vi "CleanROIs (SubVI).vi"(2 "Image Pixels (U8) 2":u8[][](array[numeric]), 3 "ROI array out 3":u32[][](array[numeric])) -> (0 "ROI array out 2":u32[][](array[numeric]))   [LabVIEW 2011, in "OfflineTracker.lvlib"]
uses:
  OfflineTracker.lvlib
panel:
  out "Array":bool[](array[boolean])
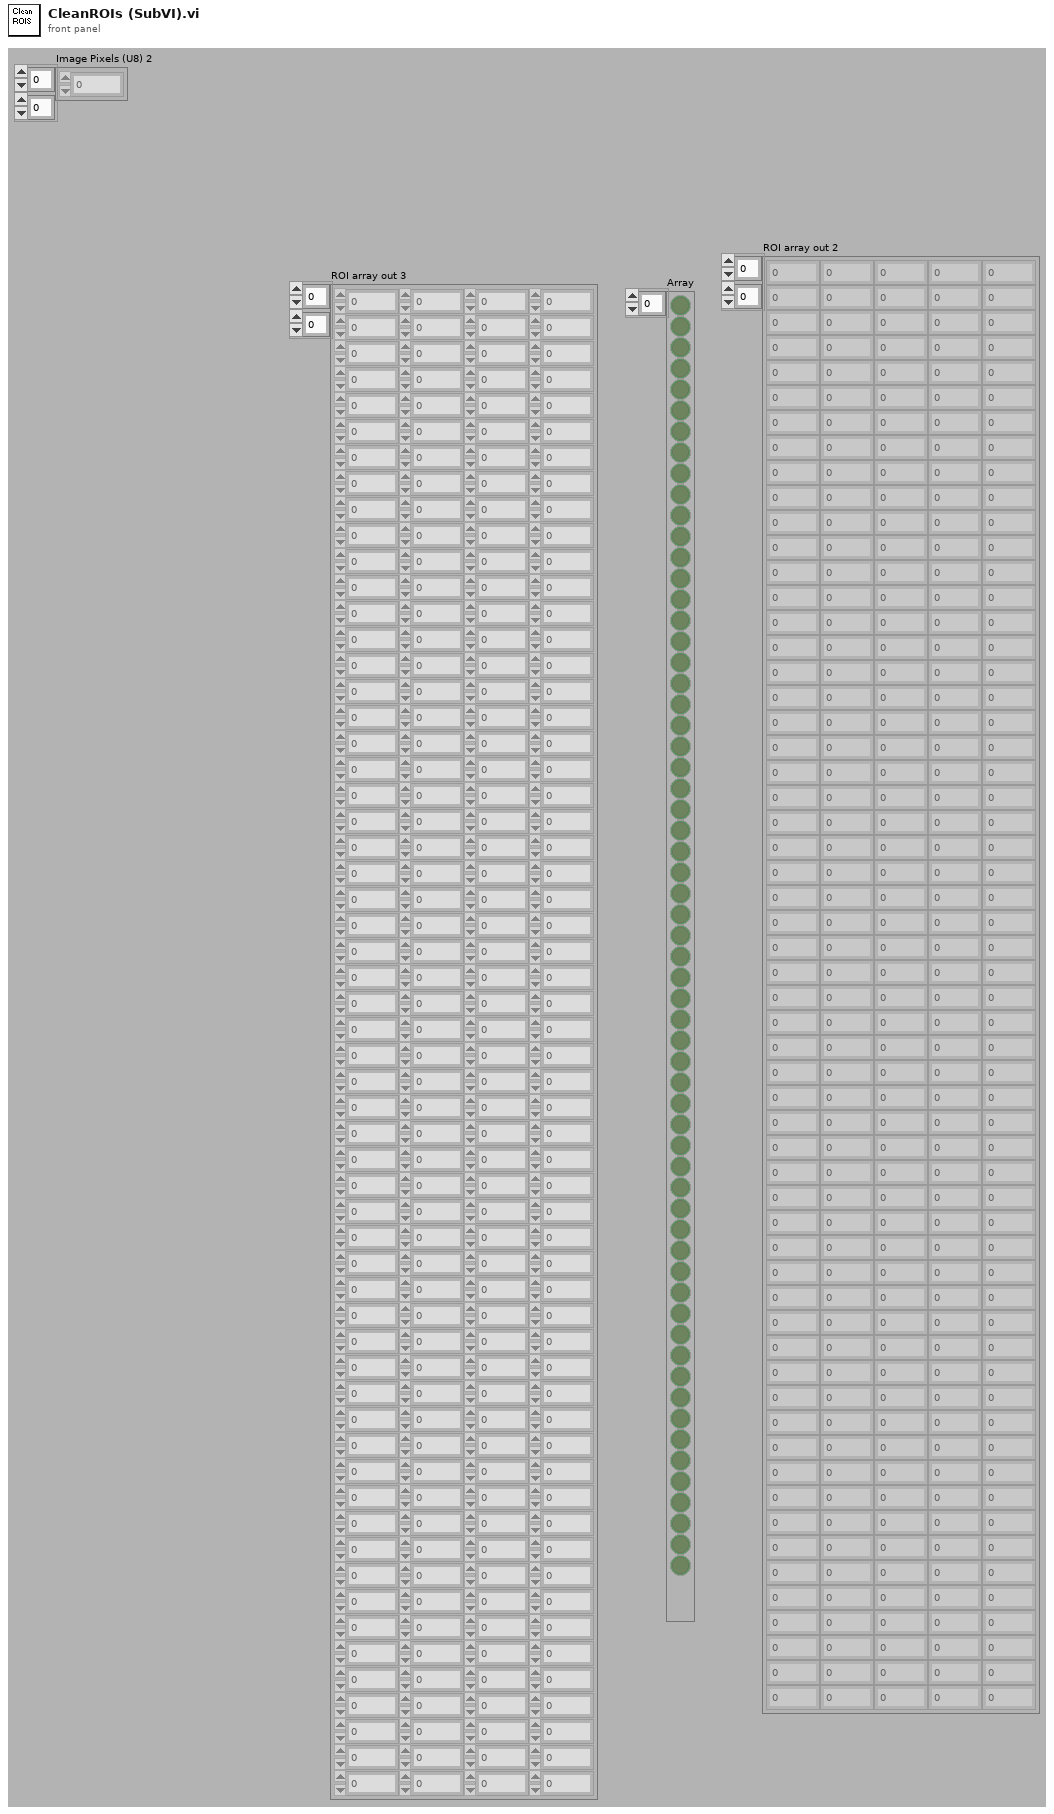
[diagram p1: front panel]
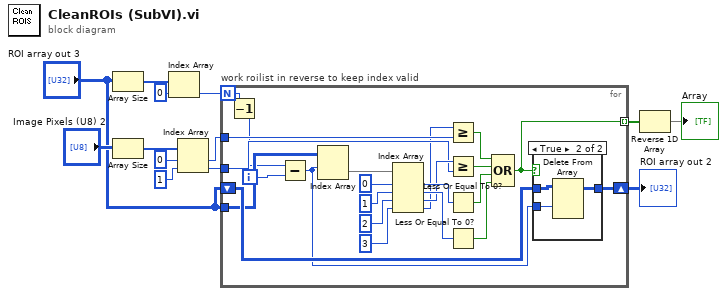
[diagram p0: block diagram]
diagram:
  n1 = Array Size(array="ROI array out 3") -> (size(s)=w6:i32[])
  n2 = Array Size(array="Image Pixels (U8) 2") -> (size(s)=w12:i32[])
  n3 = Index Array(array=w6, index=0) -> (element=w1:i32)
  n4 = Index Array(array=w12, index #1=0 ("index"), index #2=1 ("index")) -> (element #1=w9:i32, element #2=w8:i32)
  n5 = for "work roilist in reverse to keep index valid" {
    N: w1 -> [w18]
    tunnel: "ROI array out 3" -> [w21]
    tunnel: w9 -> [w30]
    tunnel: w8 -> [w31]
    tunnel: [w15] -> w3 mode=indexing
    shift-right: [w17] -> w4
    shift-left: "ROI array out 3" -> [w22]
    i -> [w19]
    n6 = Decrement(x=w18) -> (x-1=w14:i32)
    n7 = Subtract(x=w14, y=w19) -> (x-y=w16:i32)
    n8 = Index Array(array=w21, index (row)=w16) -> (element=w20:u32[])  [unwired: 1 in]
    n9 = Index Array(array=w20, index #1=0 ("index"), index #2=1 ("index"), index #3=2 ("index"), index #4=3 ("index")) -> (element #1=w34:u32, element #2=w33:u32, element #3=w32:u32, element #4=w27:u32)
    n10 = Greater Or Equal?(x=w27, y=w30) -> (x >= y?=w26:bool)
    n11 = Greater Or Equal?(x=w32, y=w31) -> (x >= y?=w25:bool)
    n12 = Less Or Equal To 0?(x=w34) -> (x <= 0?=w24:bool)
    n13 = Less Or Equal To 0?(x=w33) -> (x <= 0?=w23:bool)
    n14 = Compound Arithmetic op=OR(w26, w25, w24, w23) -> (w15:bool)
    n15 = case shown="True" w15 {
      tunnel: w22 -> [w37 w40]
      tunnel: [w37 w39] -> w17
      tunnel: w16 -> [_ w38]
      frame False {
      }
      frame True {
        n16 = Delete From Array(array=w40, index (row)=w38) -> (array with subset deleted=w39:u32[][])  [unwired: 2 in, 1 out]
      }
    }
  }
  "ROI array out 2" <- w4
  n17 = Reverse 1D Array(array=w3) -> (reversed array=→"Array":bool[])
